vi "Set Initialization Data - Acquire Data.vi"(8 "error in":errorcluster, 11 "Main View in":refnum<class "Main View.lvclass">) -> (0 "error out":errorcluster, 3 "Main View out":refnum<class "Main View.lvclass">)   [LabVIEW 2018, in "Main View.lvclass"]
doc: "Sets the initialization data of a statically linked subWorker."
uses:
  Main View.lvclass
  Acquire Data/Initialization Data.ctl
  <vilib>/addons/_Workers/Library/Classes/Message Queue/Message Queue.lvclass
  Main View.lvclass/Main View.ctl
  <vilib>/addons/_Workers/Library/Classes/Worker/Worker.lvclass/Worker.ctl
  Save Data/Save Data.lvclass
  D:/Program Files (x86)/National Instruments/LabVIEW 2018/vi.lib/addons/_Workers/Library/Classes/Worker/Worker.lvclass
  Aging View/Aging View.lvclass
  Acquire Data/Acquire Data.lvclass
  <vilib>/addons/_Workers/Library/Classes/Worker/Worker.lvclass
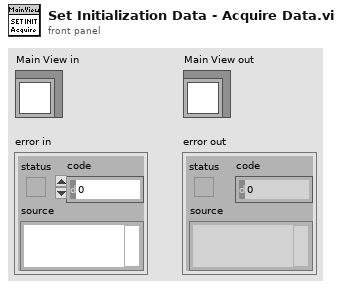
[diagram p1: front panel]
types:
  T1 = typedef "Acquire Data.lvclass/Initialization Data.ctl" = cluster{"AgingView Queue":refnum<class "Message Queue.lvclass">, "SaveData Queue":refnum<class "Message Queue.lvclass">}
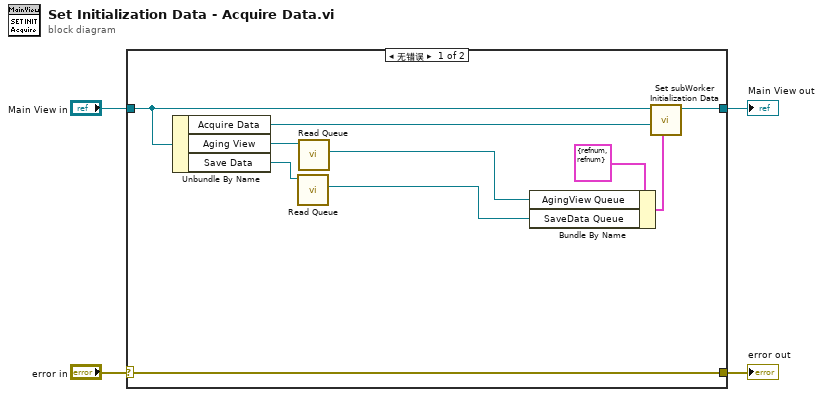
[diagram p0: block diagram]
diagram:
  n1 = case shown="无错误" "error in" {
    selector: "error in" -> [w14 w16]
    tunnel: [w14 w16] -> w3
    tunnel: [w12 w15] -> w2
    tunnel: "Main View in" -> [w11 w15]
    frame No Error {
      n2 = Unbundle By Name(w11) -> ("Acquire Data"=w13:refnum<class "Acquire Data.lvclass">, "Aging View"=w8:refnum<class "Aging View.lvclass">, "Save Data"=w7:refnum<class "Save Data.lvclass">)
      n3 = call <vilib>:"Read Queue.vi"("Worker"=w7) -> ("Message Queue out"=w5:refnum<class "Message Queue.lvclass">)  [unwired: 9 in, 1 out]
      n4 = call <vilib>:"Read Queue.vi"("Worker"=w8) -> ("Message Queue out"=w6:refnum<class "Message Queue.lvclass">)  [unwired: 9 in, 1 out]
      n5 = Bundle By Name(cluster=T1 {"AgingView Queue"=refnum, "SaveData Queue"=refnum} ("Initialization Data"), "AgingView Queue"=w6, "SaveData Queue"=w5) -> (w9:T1)
      n6 = call-dynamic "Set subWorker Initialization Data.vi"("Initialization Data"=w9, "subWorker"=w13, "Worker"=w11) -> ("Worker out"=w12:refnum<class "Main View.lvclass">)  [unwired: 8 in]
    }
    frame Error {
    }
  }
  "error out" <- w3
  "Main View out" <- w2
